vi "sweep logic test.vi"() -> ()   [LabVIEW 2017]
panel:
  out "Output":dbl
  in  "Immediate Voltage set":dbl
  in  "sweepback":bool
  in  "Voltage offset [V]":dbl
  in  "Coil Voltage Limit [V]":dbl
  in  "Immediate Voltage (V)":dbl
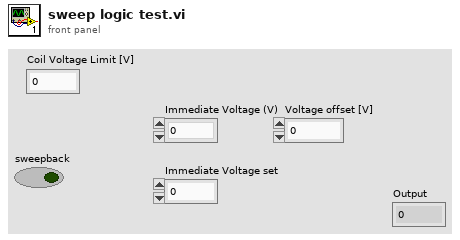
[diagram p1: front panel]
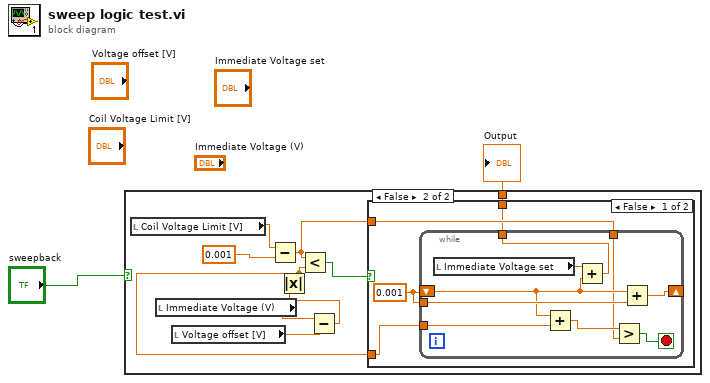
[diagram p0: block diagram]
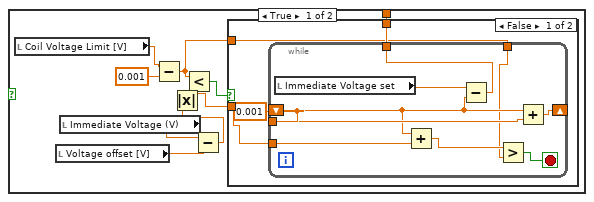
[diagram p2: hidden frame]
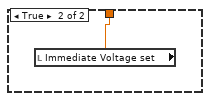
[diagram p3: hidden frame]
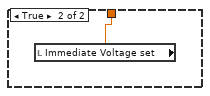
[diagram p4: hidden frame]
diagram:
  n1 = case shown="False" "sweepback" {
    tunnel: [w11 w34] -> w1
    frame True {
      n2 = local read "Coil Voltage Limit [V]"() -> (w6:dbl)
      n3 = local read "Voltage offset [V]"() -> (w9:dbl)
      n4 = local read "Immediate Voltage (V)"() -> (w10:dbl)
      n5 = Subtract(x=w6, y=0.001) -> (x-y=w4:dbl)
      n6 = Subtract(x=w10, y=w9) -> (x-y=w5:dbl)
      n7 = Absolute Value(x=w5) -> (abs(x)=w3:dbl)
      n8 = Less?(x=w4, y=w3) -> (x < y?=w8:bool)
      n9 = case shown="False" w8 {
        tunnel: [w14 w25] -> w11
        tunnel: w4 -> [w13 _]
        tunnel: w3 -> [w12 _]
        frame False {
          w15 = 0.001 ("y")
          n10 = while {
            shift-right: [w23] -> _
            shift-left: w15 -> [w19]
            tunnel: w15 -> [w22]
            tunnel: [w21] -> w14
            tunnel: w13 -> [w17]
            tunnel: w12 -> [w20]
            stop <- w24 stop-if-true
            n11 = local read "Immediate Voltage set"() -> (w16:dbl)
            n12 = Add(x=w19, y=w20) -> (x+y=w18:dbl)
            n13 = Subtract(x=w16, y=w19) -> (x-y=w21:dbl)
            n14 = Greater?(x=w18, y=w17) -> (0:w24:bool)
            n15 = Add(x=w19, y=w22) -> (x+y=w23:dbl)
          }
        }
        frame True {
          n16 = local read "Immediate Voltage set"() -> (w25:dbl)
        }
      }
    }
    frame False {
      n17 = local read "Coil Voltage Limit [V]"() -> (w29:dbl)
      n18 = local read "Immediate Voltage (V)"() -> (w33:dbl)
      n19 = local read "Voltage offset [V]"() -> (w32:dbl)
      n20 = Subtract(x=w29, y=0.001) -> (x-y=w27:dbl)
      n21 = Subtract(x=w33, y=w32) -> (x-y=w28:dbl)
      n22 = Absolute Value(x=w28) -> (abs(x)=w26:dbl)
      n23 = Less?(x=w27, y=w26) -> (x < y?=w31:bool)
      n24 = case shown="False" w31 {
        tunnel: [w36 w48] -> w34
        tunnel: w27 -> [w38 _]
        tunnel: w26 -> [w35 _]
        frame False {
          w37 = 0.001 ("y")
          n25 = while {
            shift-right: [w46] -> _
            shift-left: w37 -> [w43]
            tunnel: w38 -> [w40]
            tunnel: w37 -> [w45]
            tunnel: [w44] -> w36
            tunnel: w35 -> [w42]
            stop <- w47 stop-if-true
            n26 = local read "Immediate Voltage set"() -> (w39:dbl)
            n27 = Add(x=w43, y=w42) -> (x+y=w41:dbl)
            n28 = Add(x=w39, y=w43) -> (x+y=w44:dbl)
            n29 = Greater?(x=w41, y=w40) -> (0:w47:bool)
            n30 = Add(x=w43, y=w45) -> (x+y=w46:dbl)
          }
        }
        frame True {
          n31 = local read "Immediate Voltage set"() -> (w48:dbl)
        }
      }
    }
  }
  "Output" <- w1
